vi "Get Temp Control--Method.vi"(8 "error in (no error)":errorcluster, 11 "Simulated Thermal Process Controller in":refnum<class "Simulated Thermal Process Controller.lvclass">) -> (0 "error out":errorcluster, 1 "Output":dbl, 2 "Temp Control":bool, 3 "Simulated Thermal Process Controller out":refnum<class "Simulated Thermal Process Controller.lvclass">)   [LabVIEW 2024, in "Simulated Thermal Process Controller.lvclass"]
uses:
  Simulated Thermal Process Controller.lvclass
  Simulated Thermal Process Controller.lvclass/Simulated Thermal Process Controller.ctl
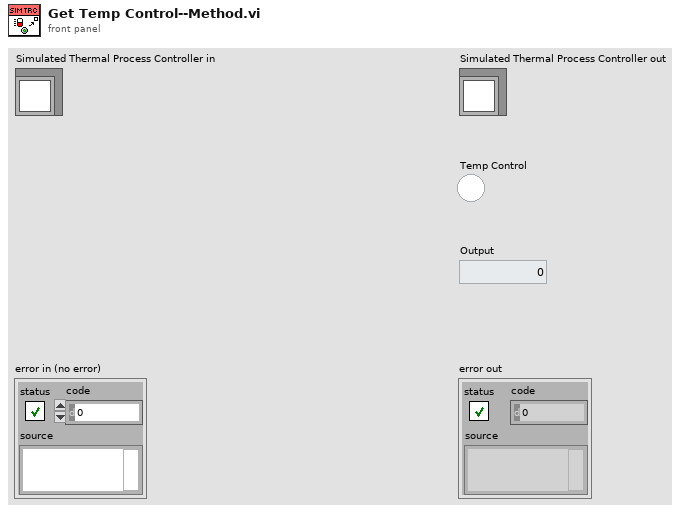
[diagram p1: front panel]
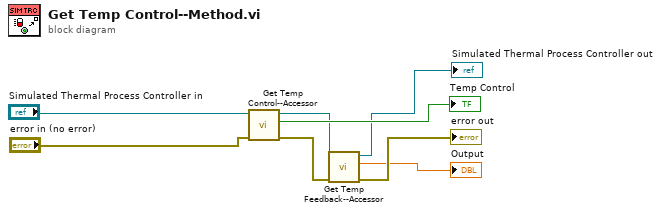
[diagram p0: block diagram]
diagram:
  n1 = call "Get Temp Control--Accessor.vi"("error in (no error)"="error in (no error)", "Simulated Thermal Process Controller in"="Simulated Thermal Process Controller in") -> ("error out"=w3:errorcluster, "Temp Control"=→"Temp Control":bool, "Simulated Thermal Process Controller out"=w5:refnum<class "Simulated Thermal Process Controller.lvclass">)  [unwired: 7 in]
  n2 = call "Get Temp Feedback--Accessor.vi"("error in (no error)"=w3, "Simulated Thermal Process Controller in"=w5) -> ("error out"=→"error out":errorcluster, "Temp Feedback"=→"Output":dbl, "Simulated Thermal Process Controller out"=→"Simulated Thermal Process Controller out":refnum<class "Simulated Thermal Process Controller.lvclass">)  [unwired: 7 in]
